vi "Read Progress.vi"(0 "HTTP GET Async handle":T1, 11 "error in (no error)":errorcluster) -> (4 "HTTP GET Async handle out":T1, 6 "file size":i64, 8 "bytes downloaded":i64, 10 "percent complete":dbl, 14 "download complete":bool, 15 "error out":errorcluster)   [LabVIEW 2019, in "HTTP Client Extensions.lvlib" / "Get Async.lvlib"]
uses:
  Get Async.lvlib
  controls/Refnum Type.ctl
  controls/Refnum Type - Enum.ctl
  GET Async.lvclass
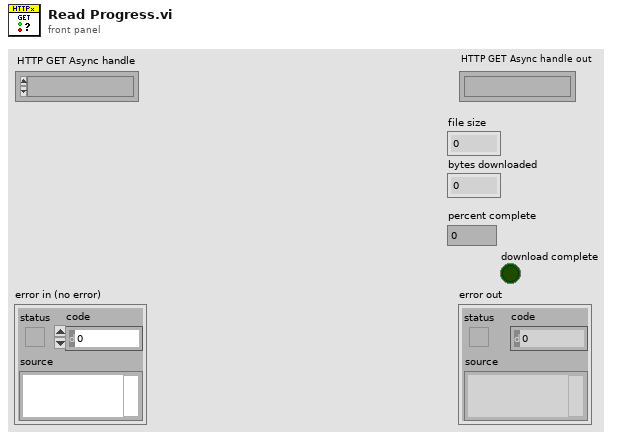
[diagram p1: front panel]
types:
  T1 = typedef "HTTP Client Extensions.lvlib/Get Async.lvlib/Refnum Type.ctl" = refnum<k1>
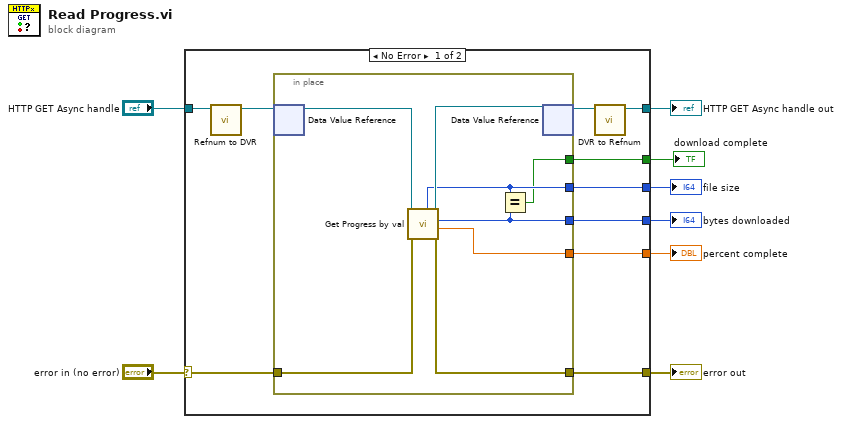
[diagram p0: block diagram]
diagram:
  n1 = case shown="No Error" "error in (no error)" {
    selector: "error in (no error)" -> [w18 w28]
    tunnel: [w17 w28] -> w7
    tunnel: [w9 w27] -> w5
    tunnel: "HTTP GET Async handle" -> [w16 w27]
    tunnel: [w12 _] -> w4
    tunnel: [w14 _] -> w3
    tunnel: [w13 _] -> w2
    tunnel: [w11 _] -> w1
    frame No Error {
      n2 = call "Refnum to DVR.vi"("Refnum out"=w16) -> ("Data Value Reference in"=w10:refnum<data-value>)  [unwired: 10 in]
      n3 = in-place {
        in-place-border: w18 -> [w25]
        in-place-border: [w22] -> w17
        in-place-border: [w20] -> w14
        in-place-border: [w24] -> w13
        in-place-border: [w21] -> w12
        in-place-border: [w19] -> w11
        n4 = in-place-dvr #1(w10) -> (w26:refnum<class "GET Async.lvclass">)  [unwired: 1 out]
        n5 = call "Get Progress by val.vi"("error in (no error)"=w25, "HTTP GET Async in"=w26) -> ("error out"=w22:errorcluster, "percent complete"=w24:dbl, "bytes downloaded"=w20:i64, "HTTP GET Async out"=w23:refnum<class "GET Async.lvclass">, "file size"=w21:i64)  [unwired: 5 in]
        n6 = Equal?(x=w21, y=w20) -> (x = y?=w19:bool)
        n7 = in-place-dvr #1(w23) -> (w15:refnum<data-value>)  [unwired: 1 out]
      }
      n8 = call "DVR to Refnum.vi"("Data Value Reference in"=w15) -> ("Refnum out"=w9:T1)  [unwired: 10 in]
    }
    frame Error {
    }
  }
  "error out" <- w7
  "HTTP GET Async handle out" <- w5
  "file size" <- w4
  "bytes downloaded" <- w3
  "percent complete" <- w2
  "download complete" <- w1
